vi "Read Port.vi"(8 "error in (no error)":errorcluster, 11 "DMD in":refnum<class "DMD.lvclass">) -> (0 "error out":errorcluster, 2 "Port":string, 3 "DMD out":refnum<class "DMD.lvclass">)   [LabVIEW 2013, in "DMD.lvclass"]
uses:
  DMD.lvclass
  DMD.lvclass/DMD.ctl
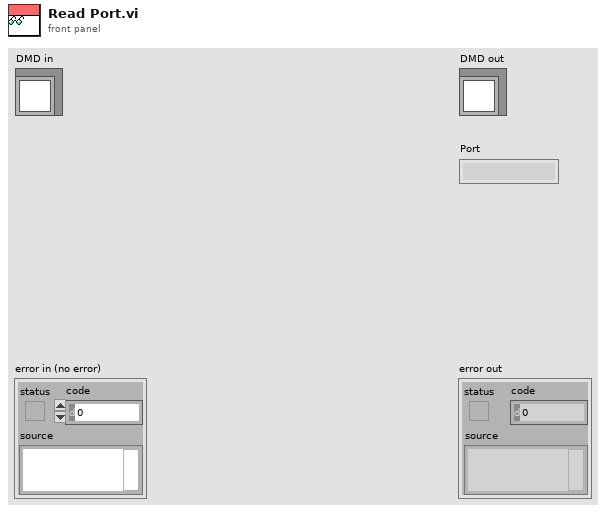
[diagram p1: front panel]
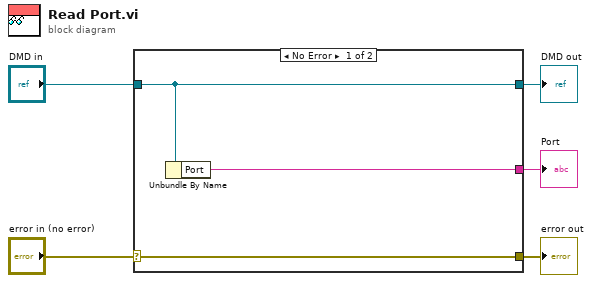
[diagram p0: block diagram]
diagram:
  n1 = case shown="No Error" "error in (no error)" {
    selector: "error in (no error)" -> [w8 w9]
    tunnel: [w8 w9] -> w4
    tunnel: [w7 w10] -> w2
    tunnel: "DMD in" -> [w7 w10]
    tunnel: [w6 _] -> w1
    frame No Error {
      n2 = Unbundle By Name(w7) -> ("Port"=w6:string)
    }
    frame Error {
    }
  }
  "error out" <- w4
  "DMD out" <- w2
  "Port" <- w1
